vi "RGB Luminosity.vi"(8 "error in (no error)":errorcluster, 9 "Blue":u8, 10 "Green":u8, 11 "Red":u8) -> (0 "error out":errorcluster, 3 "Luminosity":u8)   [LabVIEW 2018, in "Colour Lab.lvlib"]
uses:
  Colour Lab.lvlib
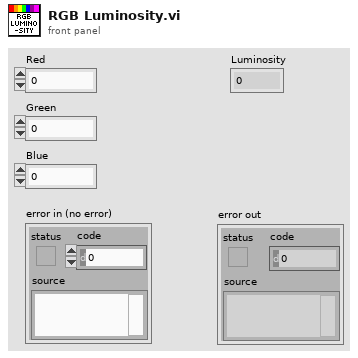
[diagram p1: front panel]
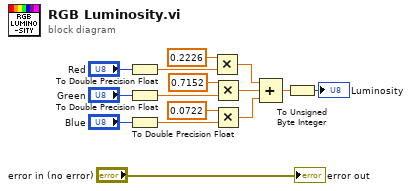
[diagram p0: block diagram]
diagram:
  n1 = To Double Precision Float(number="Red") -> (double precision float=w15:dbl)
  n2 = To Double Precision Float(number="Green") -> (double precision float=w14:dbl)
  n3 = To Double Precision Float(number="Blue") -> (double precision float=w13:dbl)
  n4 = Multiply(x=0.2226, y=w15) -> (x*y=w9:dbl)
  n5 = Multiply(x=0.7152, y=w14) -> (x*y=w8:dbl)
  n6 = Multiply(x=0.0722, y=w13) -> (x*y=w7:dbl)
  n7 = Compound Arithmetic op=ADD(w9, w8, w7) -> (w6:dbl)
  n8 = To Unsigned Byte Integer(number=w6) -> (unsigned 8bit integer=→"Luminosity":u8)
  "error out" <- "error in (no error)"
